vi "Add horizontal title.vi"(11 "path":path) -> ()   [LabVIEW 2015]
uses:
  <vilib>/Utility/file.llb/Read Delimited Spreadsheet (string).vi
  <vilib>/Utility/file.llb/Write Delimited Spreadsheet (string).vi
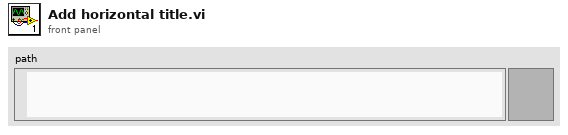
[diagram p1: front panel]
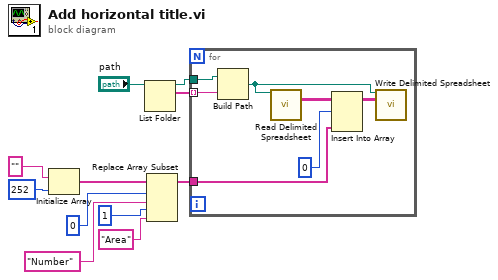
[diagram p0: block diagram]
diagram:
  n1 = Initialize Array("", 252 ("dimension size")) -> (w6:string[])
  n2 = List Folder(path="path") -> (path out=w9:path, filenames=w10:string[])  [unwired: 3 in, 2 out]
  n3 = Replace Array Subset(array=w6, new element #1="Number" ("new element/subarray"), index #1=0 ("index"), new element #2="Area" ("new element/subarray"), index #2=1 ("index")) -> (w5:string[])
  n4 = for {
    tunnel: w10 -> [w18] mode=indexing
    tunnel: w9 -> [w17]
    tunnel: w5 -> [w14]
    n5 = Build Path(base path=w17, name or relative path=w18) -> (appended path=w12:path)
    n6 = call-poly <vilib>:"Read Delimited Spreadsheet.vi"("file path (dialog if empty)"=w12) -> ("all rows"=w16:string[][])  [unwired: 9 in, 5 out]
    n7 = Insert Into Array(array=w16, index (row)=0, new element=w14) -> (w13:string[][])  [unwired: 1 in]
    n8 = call-poly <vilib>:"Write Delimited Spreadsheet.vi"("file path (dialog if empty)"=w12, "2D data"=w13) -> ()  [unwired: 12 in, 2 out]
  }
